vi "SM correction.vi"(2 "y in":dbl, 3 "x in":dbl, 4 "nm in":dbl) -> (0 "y out":dbl, 1 "x out":dbl)   [LabVIEW 2010]
panel:
  in  "Array":dbl[][](array[numeric])
  in  "Volts/pixel":dbl
  # "nmi"
  # "nmf"
  # "deltax"
  # "deltay"
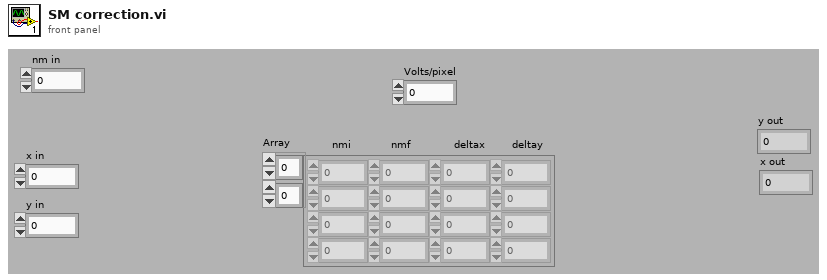
[diagram p1: front panel]
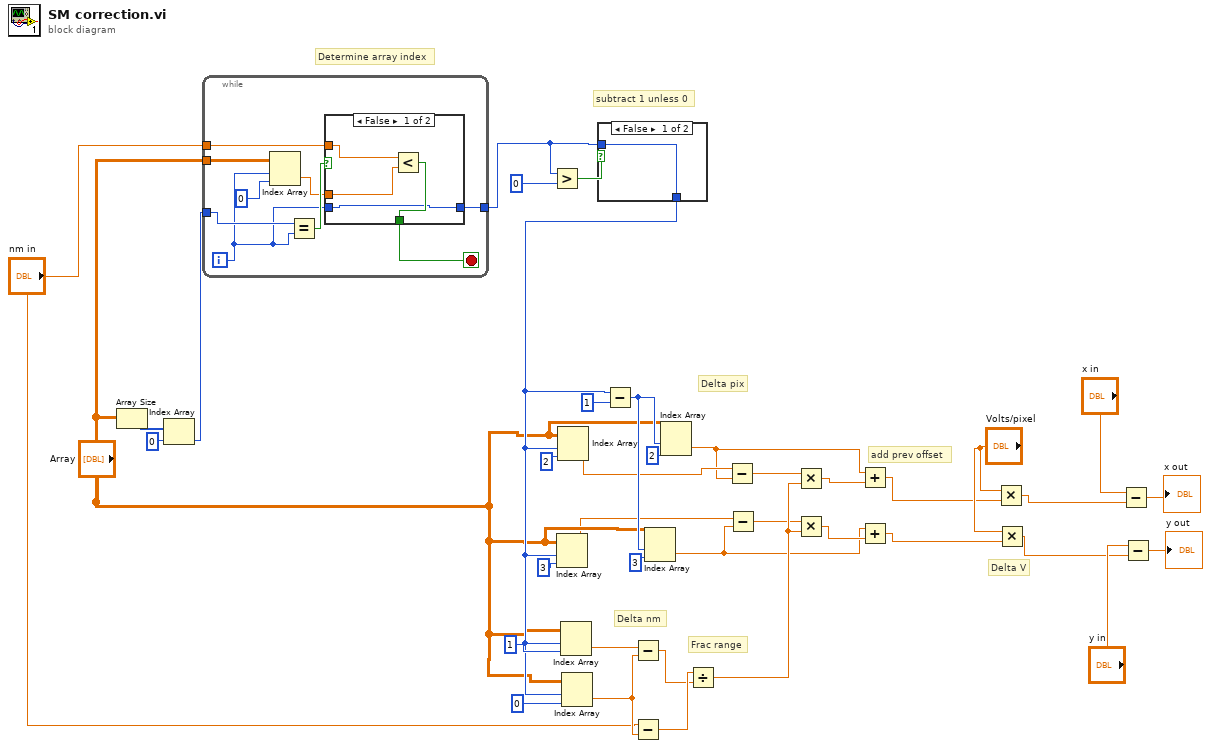
[diagram p0: block diagram]
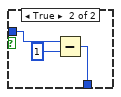
[diagram p2: hidden frame]
diagram:
  # "add prev offset"
  # "Frac range"
  # "subtract 1 unless 0"
  # "Determine array index"
  # "Delta nm"
  # "Delta V"
  # "Delta pix"
  n1 = Array Size(array="Array") -> (size(s)=w28:i32[])
  n2 = Index Array(array=w28, index=0) -> (element=w26:i32)
  n3 = while {
    tunnel: w26 -> [w46]
    tunnel: "nm in" -> [w43]
    tunnel: [w45] -> w22
    tunnel: "Array" -> [w41]
    i -> [w40]
    stop <- w44 stop-if-true
    n4 = Index Array(array=w41, index (row)=w40, index (col)=0 ("disabled index (col)")) -> (element=w42:dbl)
    n5 = Equal?(x=w46, y=w40) -> (x = y?=w47:bool)
    n6 = case shown="False" w47 {
      selector: w47 -> [_ w53]
      tunnel: w40 -> [w49 w54]
      tunnel: [w49 w54] -> w45
      tunnel: [w50 w53] -> w44
      tunnel: w43 -> [w52 _]
      tunnel: w42 -> [w51 _]
      frame False {
        n7 = Less?(x=w52, y=w51) -> (x < y?=w50:bool)
      }
      frame True {
      }
    }
  }
  n8 = Greater?(x=w22, y=0) -> (0:w23:bool)
  n9 = case shown="False" w23 {
    tunnel: w22 -> [w55 w58]
    tunnel: [w55 w56] -> w19
    frame False {
    }
    frame True {
      n10 = Subtract(x=w58, y=1) -> (x-y=w56:i32)
    }
  }
  n11 = Index Array(array="Array", index (row)=w19, index (col)=3 ("index")) -> (element=w12:dbl)
  n12 = Index Array(array="Array", index (row)=w19, index (col)=2 ("index")) -> (element=w13:dbl)
  n13 = Index Array(array="Array", index (row)=w19, index (col)=1 ("index")) -> (element=w34:dbl)
  n14 = Index Array(array="Array", index (row)=w19, index (col)=0 ("index")) -> (element=w29:dbl)
  n15 = Subtract(x=w19, y=1) -> (x-y=w17:i32)
  n16 = Subtract(x=w34, y=w29) -> (x-y=w20:dbl)
  n17 = Subtract(x="nm in", y=w29) -> (x-y=w21:dbl)
  n18 = Index Array(array="Array", index (row)=w17, index (col)=3) -> (element=w6:dbl)
  n19 = Index Array(array="Array", index (row)=w17, index (col)=2) -> (element=w5:dbl)
  n20 = Divide(x=w21, y=w20) -> (x/y=w11:dbl)
  n21 = Subtract(x=w13, y=w5) -> (x-y=w10:dbl)
  n22 = Subtract(x=w12, y=w6) -> (x-y=w9:dbl)
  n23 = Multiply(x=w10, y=w11) -> (x*y=w8:dbl)
  n24 = Multiply(x=w9, y=w11) -> (x*y=w7:dbl)
  n25 = Add(x=w5, y=w8) -> (x+y=w2:dbl)
  n26 = Add(x=w6, y=w7) -> (x+y=w1:dbl)
  n27 = Multiply(x="Volts/pixel", y=w2) -> (x*y=w4:dbl)
  n28 = Multiply(x="Volts/pixel", y=w1) -> (x*y=w3:dbl)
  n29 = Subtract(x="x in", y=w4) -> (x-y=→"x out":dbl)
  n30 = Subtract(x="y in", y=w3) -> (x-y=→"y out":dbl)
